vi "Convert_Into_SI_Units.vi"(6 "Microsteps (MS=64)":dbl=64.0, 7 "Motor":u16(ring) items=["none", "1", "2", "3", "4", "all"], 8 "Input Unit":T1=enum."Meter", 10 "Input":dbl) -> (2 "Output":dbl)   [LabVIEW 2013]
uses:
  Unit_Control.ctl
  Constants.ctl
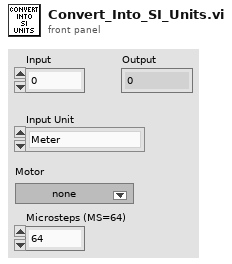
[diagram p1: front panel]
types:
  T1 = typedef "Unit_Control.ctl" = enum16{"Angle (Degrees)", "Rad", "Angle [TMC]", "Microsteps [TMC]", "Inches", "Nanometer", "Meter", "Centimeter", "Millimeter", "Micron", "Joule", "Electron Volts", "Hertz", "Terahertz", "Megahertz"}
  T2 = typedef "Constants.ctl" = dbl
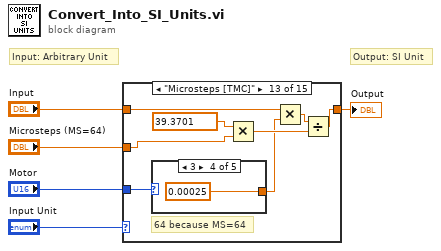
[diagram p0: block diagram]
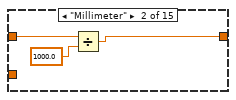
[diagram p3: hidden frame]
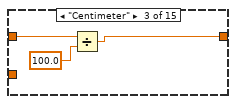
[diagram p4: hidden frame]
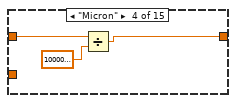
[diagram p5: hidden frame]
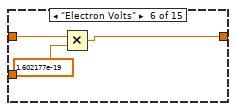
[diagram p7: hidden frame]
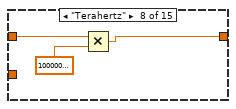
[diagram p9: hidden frame]
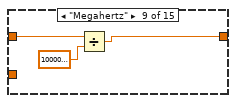
[diagram p10: hidden frame]
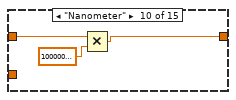
[diagram p11: hidden frame]
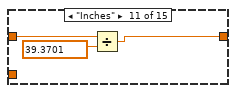
[diagram p12: hidden frame]
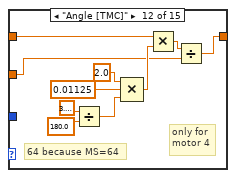
[diagram p13: hidden frame]
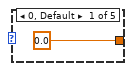
[diagram p14: hidden frame]
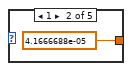
[diagram p15: hidden frame]
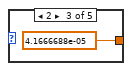
[diagram p16: hidden frame]
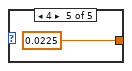
[diagram p17: hidden frame]
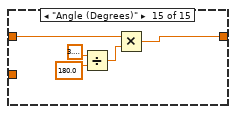
[diagram p19: hidden frame]
diagram:
  # "Output: SI Unit"
  # "Input: Arbitrary Unit"
  n1 = case shown="\"Microsteps [TMC]\"" "Input Unit" {
    tunnel: "Input" -> [w6 w9 w12 w15 w16 w19 w20 w23 w26 w29 w31 w41 w47 w56 w59]
    tunnel: [w6 w8 w10 w14 w16 w18 w20 w22 w25 w27 w30 w40 w46 w56 w57] -> w5
    tunnel: "Motor" -> [_ _ _ _ _ _ _ _ _ _ _ _ w45 _ _]
    tunnel: "Microsteps (MS=64)" -> [_ _ _ _ _ _ _ _ _ _ _ w33 w44 _ _]
    frame "Meter", Default {
    }
    frame "Millimeter" {
      n2 = Divide(x=w9, y=1000.0) -> (x/y=w8:dbl)
    }
    frame "Centimeter" {
      n3 = Divide(x=w12, y=100.0) -> (x/y=w10:dbl)
    }
    frame "Micron" {
      n4 = Divide(x=w15, y=1000000.0) -> (x/y=w14:dbl)
    }
    frame "Joule" {
    }
    frame "Electron Volts" {
      w17 = T2 1.602177e-19 items=["pi (Number)"=3.141593, "e [As]"=1.602177e-19, "h [Js]"=6.62607e-34, "c [m/s]"=299792500.0, "e (Number)"=2.718282] ("Constants")
      n5 = Multiply(x=w19, y=w17) -> (x*y=w18:T2)
    }
    frame "Hertz" {
    }
    frame "Terahertz" {
      n6 = Multiply(x=w23, y=1000000000000.0) -> (x*y=w22:dbl)
    }
    frame "Megahertz" {
      n7 = Divide(x=w26, y=1000000.0) -> (x/y=w25:dbl)
    }
    frame "Nanometer" {
      n8 = Multiply(x=w29, y=1000000000000.0) -> (x*y=w27:dbl)
    }
    frame "Inches" {
      n9 = Divide(x=w31, y=39.3701) -> (x/y=w30:dbl)
    }
    frame "Angle [TMC]" {
      # "only for\nmotor 4"
      # "64 because MS=64"
      n10 = Divide(x=3.141592653589793, y=180.0) -> (x/y=w35:dbl)
      n11 = Compound Arithmetic op=MULTIPLY(2.0 ("x"), 0.01125, w35) -> (w34:dbl)
      n12 = Multiply(x=w41, y=w34) -> (x*y=w42:dbl)
      n13 = Divide(x=w42, y=w33) -> (x/y=w40:dbl)
    }
    frame "Microsteps [TMC]" {
      # "64 because MS=64"
      n14 = case shown="3" w45 {
        tunnel: [0.0 4.1666688e-05 4.1666688e-05 0.00025 0.0225] -> w43
        frame 0, Default {
        }
        frame 1 {
        }
        frame 2 {
        }
        frame 3 {
        }
        frame 4 {
        }
      }
      n15 = Multiply(x=39.3701, y=w44) -> (x*y=w48:dbl)
      n16 = Multiply(x=w47, y=w43) -> (x*y=w50:dbl)
      n17 = Divide(x=w50, y=w48) -> (x/y=w46:dbl)
    }
    frame "Rad" {
    }
    frame "Angle (Degrees)" {
      n18 = Divide(x=3.141592653589793, y=180.0) -> (x/y=w58:dbl)
      n19 = Multiply(x=w59, y=w58) -> (x*y=w57:dbl)
    }
  }
  "Output" <- w5
